vi "Arduino_Check_Main_v1.vi"() -> ()   [LabVIEW 2021]
uses:
  Drivers/Arduino_Pulse_Generator/Configurate/Channel_Pulse_Stream.ctl
  Drivers/Arduino_Pulse_Generator/Configurate/Register_1.ctl
  Drivers/Arduino_Pulse_Generator/Configurate/Register_2.ctl
panel:
  out "register 2 (8-13)":T1
  out "register 1 (2-7)":T2
  out "Pulse sequence":T3[](array[typedef]) {"channel" min=2 max=13 step=1}
  out "error out":errorcluster
  in  "error in":errorcluster
  in  "VISA arduino in":refnum<visa-resource-name>
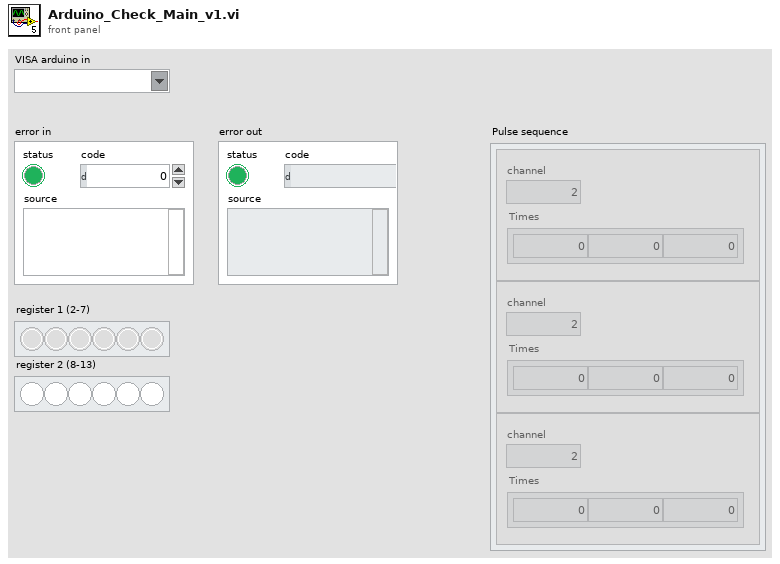
[diagram p1: front panel]
types:
  T1 = typedef "Register_2.ctl" = bool[]
  T2 = typedef "Register_1.ctl" = bool[]
  T3 = typedef "Channel_Pulse_Stream.ctl" = cluster{"Times":dbl[], "channel":u8}
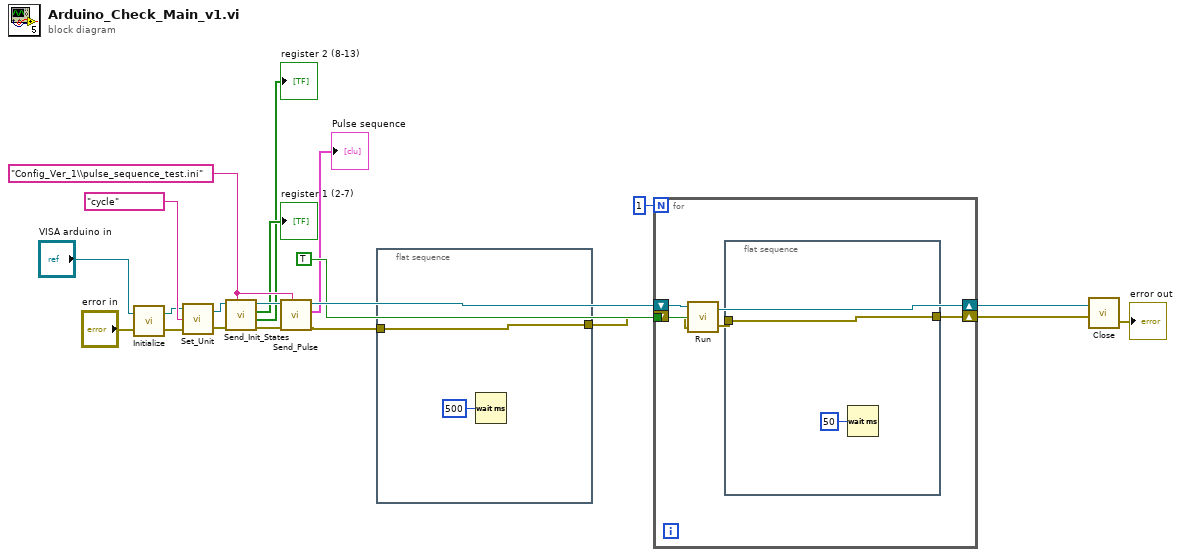
[diagram p0: block diagram]
diagram:
  w17 = "Config_Ver_1\\pulse_sequence_test.ini" ("Filename (.ini)")
  n1 = call "Initialize.vi"("error in"="error in", "VISA arduino in"="VISA arduino in") -> ("error out"=w12:errorcluster, "VISA arduino out"=w11:refnum<visa-resource-name>)
  n2 = call "Set_Unit.vi"("error in"=w12, "Unit"="cycle", "VISA arduino in"=w11) -> ("error out"=w14:errorcluster, "VISA arduino out"=w15:refnum<visa-resource-name>)
  n3 = call "Send_Init_States.vi"("Filename (.ini)"=w17, "error in"=w14, "VISA arduino in"=w15) -> ("error out"=w18:errorcluster, "register 2 (8-13)"=→"register 2 (8-13)":T1, "register 1 (2-7)"=→"register 1 (2-7)":T2, "VISA arduino out"=w19:refnum<visa-resource-name>)  [unwired: 5 in]
  n4 = call "Send_Pulse.vi"("Filename (.ini)"=w17, "error in"=w18, "VISA arduino in"=w19) -> ("error out"=w3:errorcluster, "Pulse sequence"=→"Pulse sequence":T3[], "VISA arduino out"=w16:refnum<visa-resource-name>)  [unwired: 6 in]
  n5 = flat-sequence {
    tunnel: [w23] -> w4
    tunnel: w3 -> [w23]
    frame #0 {
      n6 = Wait (ms)(milliseconds to wait=u32 500) -> ()  [unwired: 1 out]
    }
  }
  n7 = for {
    N: 1 -> [_]
    tunnel: TRUE ("run?") -> [w28]
    shift-right: [w27] -> w9
    shift-left: w16 -> [w29]
    shift-right: [w24] -> w2
    shift-left: w4 -> [w26]
    n8 = call "Run.vi"("error in"=w26, "run?"=w28, "VISA arduino in"=w29) -> ("error out"=w25:errorcluster, "VISA arduino out"=w27:refnum<visa-resource-name>)
    n9 = flat-sequence {
      tunnel: [w31] -> w24
      tunnel: w25 -> [w31]
      frame #0 {
        n10 = Wait (ms)(milliseconds to wait=u32 50) -> ()  [unwired: 1 out]
      }
    }
  }
  n11 = call "Close.vi"("error in"=w2, "VISA arduino in"=w9) -> ("error out"=→"error out":errorcluster)  [unwired: 1 in]
